vi "updateMTStandard.vi"() -> ()   [LabVIEW 2012]
uses:
  <vilib>/addons/database/Connection.llb/DB Tools Open Connec (Path).vi
  <vilib>/addons/database/Connection.llb/Conn Execute.vi
  <vilib>/addons/database/Recordset.llb/Rec Destroy - Connection.vi
  <vilib>/addons/database/NI_Database_API.lvlib
panel:
  out "error out":errorcluster
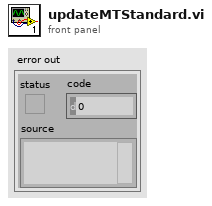
[diagram p1: front panel]
types:
  T1 = typedef "NI_Database_API.lvlib/Conn ObjectReference.ctl" = refnum<k1>
  T2 = typedef "NI_Database_API.lvlib/Rec ObjectReference.ctl" = refnum<k1>
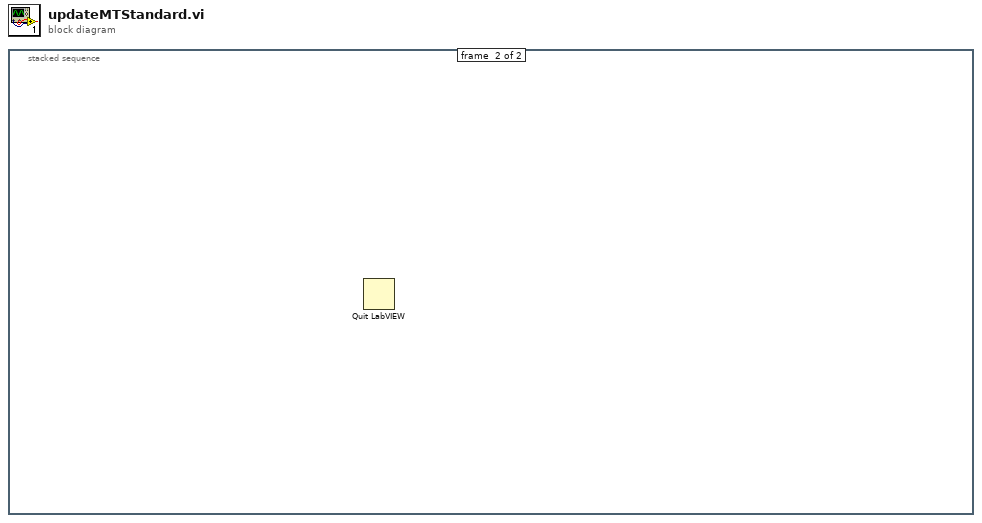
[diagram p0: block diagram]
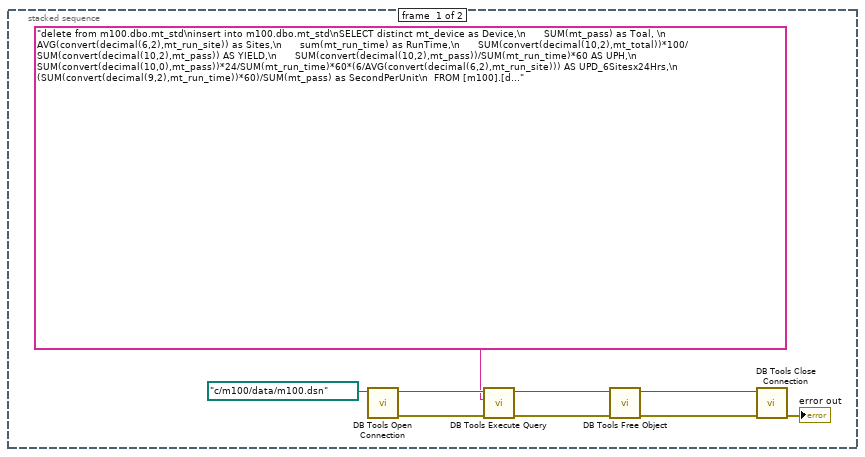
[diagram p2: hidden frame]
diagram:
  n1 = stacked-sequence {
    frame #0 {
      n2 = call-poly <vilib>:"DB Tools Open Connection.vi"("connection information"=path "c:/m100/data/m100.dsn") -> ("error out"=w6:errorcluster, "connection reference"=w9:T1)  [unwired: 7 in]
      n3 = call-poly <vilib>:"DB Tools Execute Query.vi"("error in (no error)"=w6, "SQL query"="delete from m100.dbo.mt_std\ninsert into m100.dbo.mt_std\nSELECT distinct mt_device as Device,\n      SUM(mt_pass) as Toal, \n      AVG(convert(decimal(6,2),mt_run_site)) as Sites,\n      sum(mt_run_time) as RunTime,\n      SUM(convert(decimal(10,2),mt_total))*100/SUM(convert(decimal(10,2),mt_pass)) AS YIELD,\n      SUM(convert(decimal(10,2),mt_pass))/SUM(mt_run_time)*60 AS UPH,\n      SUM(convert(decimal(10,0),mt_pass))*24/SUM(mt_run_time)*60*(6/AVG(convert(decimal(6,2),mt_run_site))) AS UPD_6Sitesx24Hrs,\n      (SUM(convert(decimal(9,2),mt_run_time))*60)/SUM(mt_pass) as SecondPerUnit\n  FROM [m100].[dbo].[mt_data] with (Nolock)\n  where mt_date between convert(varchar, getdate()-30, 111) and convert(varchar, getdate(), 111)\n    and mt_pass > 10\n    and mt_device <> ''\n    and mt_package <> ''\n    and mt_run_time=60\n    and mt_run_site=6\n    and mt_file like '%MT%'\n  group by mt_device\n  order by mt_device", "connection reference"=w9) -> ("error out"=w5:errorcluster, "recordset reference"=w8:T2)  [unwired: 5 in]
      n4 = call-poly <vilib>:"DB Tools Free Object.vi"("error in (no error)"=w5, "recordset reference"=w8) -> ("error out"=w4:errorcluster, "connection reference"=w7:T1)  [unwired: 8 in]
      n5 = call <vilib>:"DB Tools Close Connection.vi"("error in (no error)"=w4, "connection reference"=w7) -> ("error out"=→"error out":errorcluster)  [unwired: 5 in]
    }
    frame #1 {
      n6 = Quit LabVIEW() -> ()  [unwired: 1 in]
    }
  }
